vi "Get Variant.vi"(8 "error in (no error)":errorcluster, 11 "Message in":refnum<class "Raw Message.lvclass">) -> (0 "error out":errorcluster, 2 "Variant":variant, 3 "Message out":refnum<class "Raw Message.lvclass">)   [LabVIEW 2020, in "Protobuf RAW.lvlib" / "Raw Message.lvclass"]
uses:
  Raw Message.lvclass
  Raw Message.lvclass/Raw Message.ctl
  Tag/Basic Type.lvclass
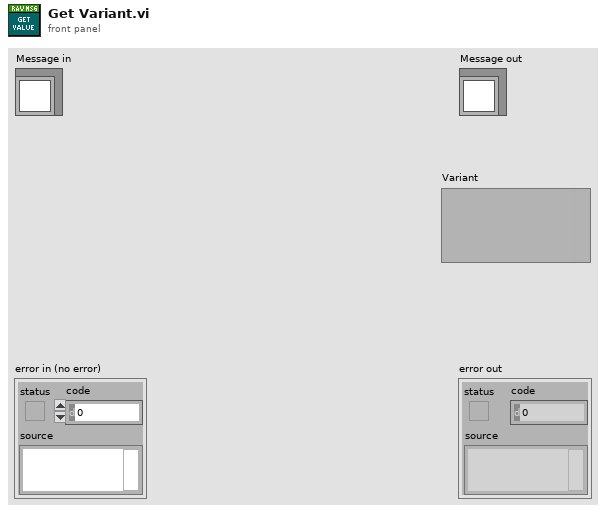
[diagram p1: front panel]
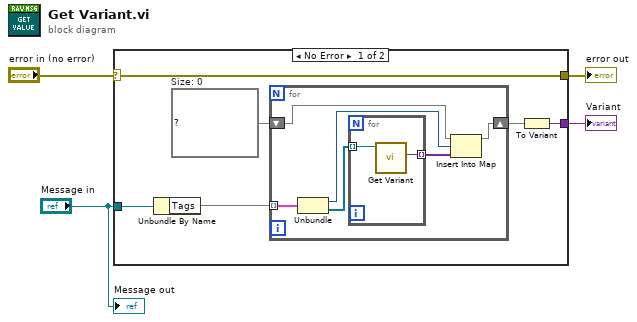
[diagram p0: block diagram]
diagram:
  n1 = case shown="No Error" "error in (no error)" {
    selector: "error in (no error)" -> [w6 w19]
    tunnel: "Message in" -> [w10 _]
    tunnel: [w5 _] -> w3
    tunnel: [w6 w19] -> w1
    frame No Error {
      w7 = map{u32, variant[]} {}  # Size: 0
      n2 = Unbundle By Name(w10) -> ("Tags"=w9:map{u32, refnum<class "Basic Type.lvclass">[]})
      n3 = for {
        tunnel: w9 -> [w16] mode=indexing
        shift-right: [w13] -> w8
        shift-left: w7 -> [w14]
        n4 = Unbundle(w16) -> ("ID"=w12:u32, "Tag"=w15:refnum<class "Basic Type.lvclass">[])
        n5 = for {
          tunnel: w15 -> [w18] mode=indexing
          tunnel: [w17] -> w11 mode=indexing
          n6 = call-dynamic "Get Variant.vi"("Type Serializer in"=w18) -> ("Variant"=w17:variant)  [unwired: 8 in, 2 out]
        }
        n7 = Insert Into Map(map in=w14, key=w12, value=w11) -> (map out=w13:map{u32, variant[]})  [unwired: 2 out]
      }
      n8 = To Variant(anything=w8) -> (Variant=w5:variant)
    }
    frame Error {
    }
  }
  "error out" <- w1
  "Variant" <- w3
  "Message out" <- "Message in"
